vi "Save Scores.vi"(8 "error in (no error)":errorcluster, 9 "Test Summary":string, 10 "Score":T1, 11 "LLB Path":path) -> (0 "error out":errorcluster)   [LabVIEW 2020]
uses:
  <vilib>/Utility/config.llb/Write Key (Double).vi
  <vilib>/Utility/config.llb/Write Key (String).vi
  <vilib>/Utility/config.llb/Write Key (I32).vi
  <vilib>/Utility/config.llb/NI_LVConfig.lvlib
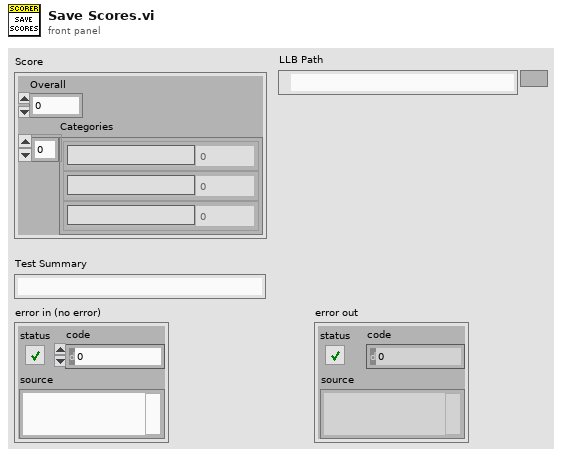
[diagram p1: front panel]
types:
  T1 = cluster{"Overall":dbl, "Categories":cluster{"Category":string, "Value":dbl}[]}
  T2 = typedef "NI_LVConfig.lvlib/Config Data RefNum.ctl" = refnum<k1>
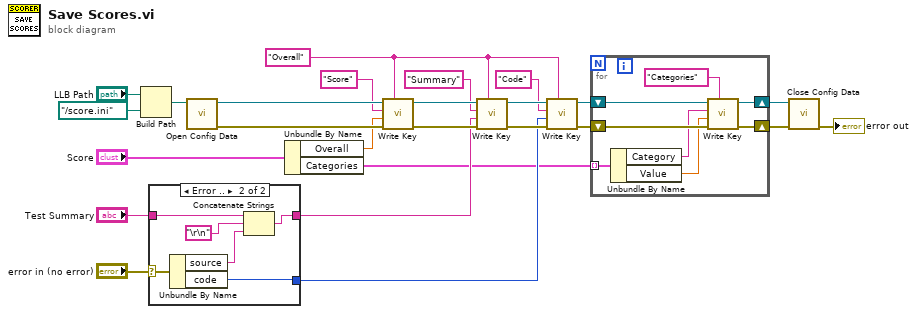
[diagram p0: block diagram]
diagram:
  w9 = "Overall" ("section")
  n1 = Build Path(base path="LLB Path", name or relative path=path "../score.ini") -> (appended path=w23:path)
  n2 = case shown="Error .." "error in (no error)" {
    selector: "error in (no error)" -> [_ w30]
    tunnel: "Test Summary" -> [w26 w32]
    tunnel: [w26 w28] -> w12
    tunnel: [_ w27] -> w7
    frame No Error {
    }
    frame Error {
      n3 = Unbundle By Name(w30) -> ("source"=w29:string, "code"=w27:i32)
      n4 = Concatenate Strings(w32, "\r\n", w29) -> (w28:string)
    }
  }
  n5 = call <vilib>:"Open Config Data.vi"("configuration file path"=w23) -> ("error out"=w16:errorcluster, "refnum"=w20:T2)  [unwired: 8 in, 1 out]
  n6 = Unbundle By Name("Score") -> ("Overall"=w14:dbl, "Categories"=w4:cluster{"Category":string, "Value":dbl}[])
  n7 = call-poly <vilib>:"Write Key.vi"("section"=w9, "error in (no error)"=w16, "value"=w14, "key"="Score", "refnum"=w20) -> ("error out"=w15:errorcluster, "refnum out"=w18:T2)  [unwired: 4 in, 1 out]
  n8 = call-poly <vilib>:"Write Key.vi"("section"=w9, "error in (no error)"=w15, "value"=w12, "key"="Summary", "refnum"=w18) -> ("error out"=w10:errorcluster, "refnum out"=w11:T2)  [unwired: 4 in, 1 out]
  n9 = call-poly <vilib>:"Write Key.vi"("section"=w9, "error in (no error)"=w10, "value"=w7, "key"="Code", "refnum"=w11) -> ("error out"=w5:errorcluster, "refnum out"=w6:T2)  [unwired: 4 in, 1 out]
  n10 = for {
    shift-right: [w34] -> w3
    shift-left: w6 -> [w40]
    shift-right: [w33] -> w2
    shift-left: w5 -> [w38]
    tunnel: w4 -> [w37] mode=indexing
    n11 = Unbundle By Name(w37) -> ("Category"=w36:string, "Value"=w35:dbl)
    n12 = call-poly <vilib>:"Write Key.vi"("section"="Categories", "error in (no error)"=w38, "value"=w35, "key"=w36, "refnum"=w40) -> ("error out"=w33:errorcluster, "refnum out"=w34:T2)  [unwired: 4 in, 1 out]
  }
  n13 = call <vilib>:"Close Config Data.vi"("error in (no error)"=w2, "refnum"=w3) -> ("error out"=→"error out":errorcluster)  [unwired: 8 in, 1 out]
